vi "BackgroundFulltrackCalculations_171213.vi"(6 "360Y":dbl[](array[numeric]), 7 "Mousebackground":picture, 9 "360X":dbl[](array[numeric]), 10 "ForAnalysisLastRecordingPath":path, 11 "Slide in":refnum<vi>) -> (1 "BackgroundSegmentforAnalysis":picture, 2 "NormalMousebackgroundOutput":picture, 3 "BackgroundSegmentsOutput":picture, 4 "HeatMap":dbl[][](array[numeric]))   [LabVIEW 2016]
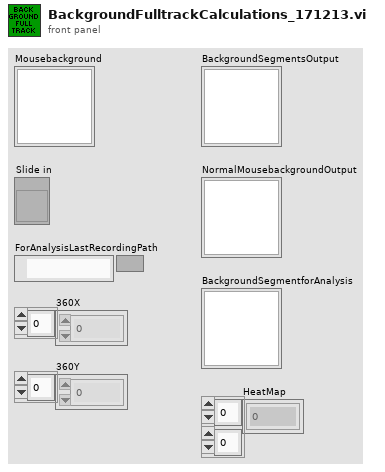
[diagram p1: front panel]
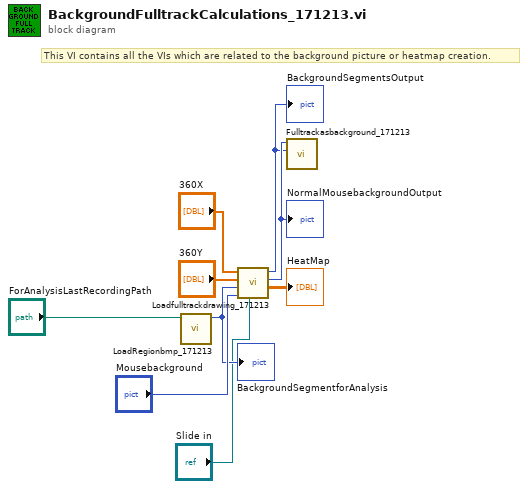
[diagram p0: block diagram]
diagram:
  # "This VI contains all the VIs which are related to the background picture or heatmap creation."
  n1 = call "LoadRegionbmp_171213.vi"("SelectedPath"="ForAnalysisLastRecordingPath") -> ("BackgroundSegmentforAnalysis"=w3:picture)  [unwired: 10 in]
  "BackgroundSegmentforAnalysis" <- w3
  n2 = call "Loadfulltrackdrawing_171213.vi"("Slide in 2"="Slide in", "NormalMouseBackgroundInput"="Mousebackground", "BackgroundSegmentsInput"=w3, "360Y"="360Y", "360X"="360X") -> ("HeatMap"=→"HeatMap":dbl[][], "NormalMousebackgroundOutput"=w7:picture, "BackgroundSegmentsOutput"=w6:picture)  [unwired: 4 in]
  "NormalMousebackgroundOutput" <- w7
  "BackgroundSegmentsOutput" <- w6
  n3 = call "Fulltrackasbackground_171213.vi"("FullTracakonSegments"=w6, "FullTrackonNormalMouseBackground"=w7) -> ()  [unwired: 10 in]
